vi "array2ColVector.vi"(1 "vector":dbl[](array[numeric])) -> (0 "col vector":dbl[][](array[numeric]))   [LabVIEW 2017, in "NI_Gmath.lvlib"]
uses:
  <vilib>/gmath/NI_Gmath.lvlib
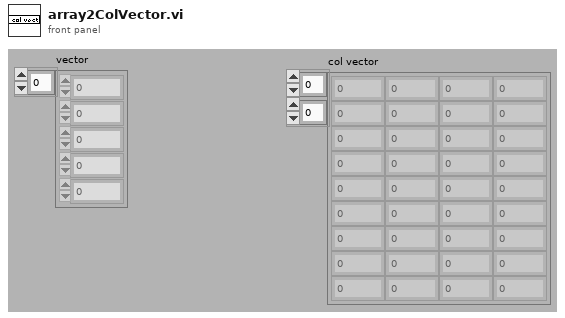
[diagram p1: front panel]
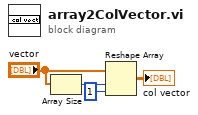
[diagram p0: block diagram]
diagram:
  n1 = Array Size(array="vector") -> (size(s)=w2:i32)
  n2 = Reshape Array("vector", w2, 1 ("dimension size")) -> (→"col vector":dbl[][])
